vi "BotSpeak.BaseCom.vi"(3 "Termination":string="\r\n", 5 "command":string="PING", 6 "Bot Settings in":T1) -> (0 "response":string="169.254.32.85", 2 "Bot Settings out":T1)   [LabVIEW 2014]
doc: "Protocol:\nLCD \"text to write\" 0,0 // start row, start col (0,0 default)\nBTN // replies with a 5 bit number bot PB1-PB5\nLED 64 // each bit corresponds to an LED\nAI 0 // replies with the value of A/D 0\nAO 2.5,1.34 // sets DAC 0 to 2.5 v and DAC 1 to 1.34 v\nDIO 3,1 // sets DIO 3 to HIGH\nDIO 3 // reads DIO 3 and returns state\nIP // returns IP Address\nTEMP // returns Temperature reading"
uses:
  <userlib>/botspeakLib/VIs/Direct/BotSpeak_Control.ctl
  <userlib>/botspeakLib/VIs/SubVIs/BotSpeak_Globals.vi
panel:
  # "GET DIO[DIO[1]}"
  # "to do:\n\n\nAbort does not work."
  # "use Address \"close\" to close the \nlast connection"
  # "blank means no reply"
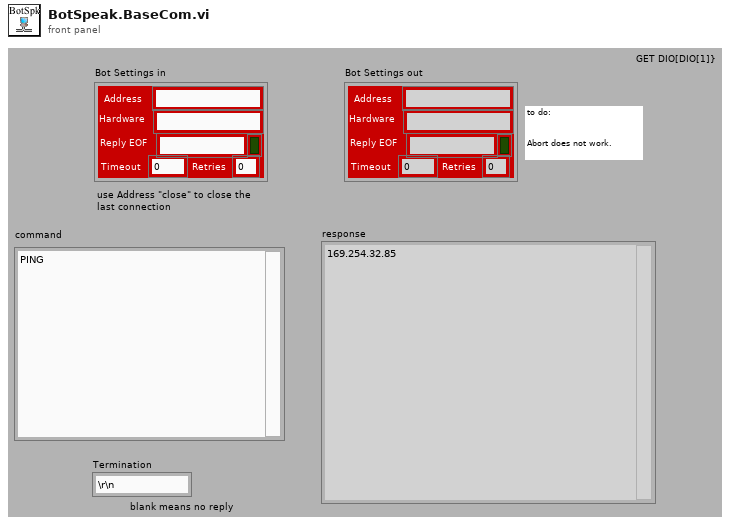
[diagram p1: front panel]
types:
  T1 = typedef "BotSpeak_Control.ctl" = cluster{"Address":string, "Reply EOF":string, "Hardware":string, "Retries":i8, "Timeout":i32, "Open?":bool}
  T2 = typedef "CommState.ctl" = cluster{"Bot Settings":T1, "Initialized":bool, "Talking":bool}
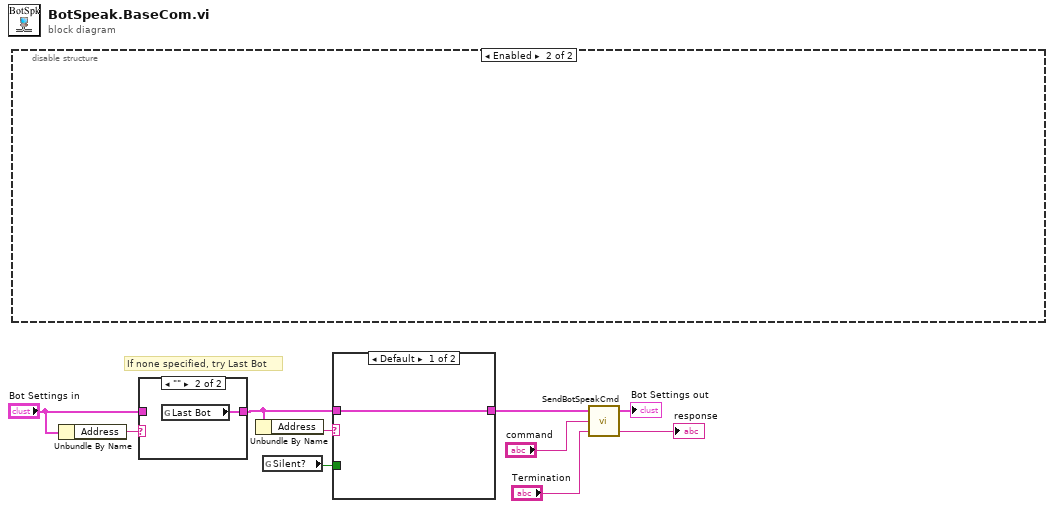
[diagram p0: block diagram]
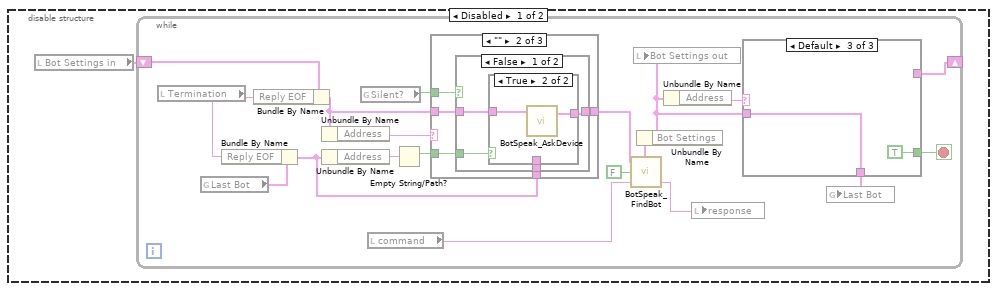
[diagram p2: hidden frame]
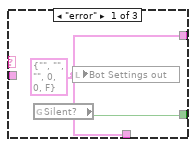
[diagram p3: hidden frame]
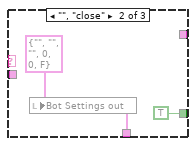
[diagram p4: hidden frame]
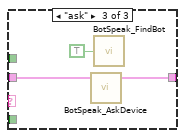
[diagram p8: hidden frame]
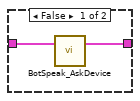
[diagram p10: hidden frame]
diagram:
  # "If none specified, try Last Bot"
  n1 = disable-structure shown="Enabled" {
    frame Disabled {
      n2 = local read "Bot Settings in"() -> (w11:T1)
      n3 = while {
        shift-right: [w17] -> _
        shift-left: w11 -> [w18]
        stop <- w19 stop-if-true
        n4 = local read "Termination"() -> (w15:string)
        n5 = global read "BotSpeak_Globals.vi" "Last Bot"() -> (w24:T1)
        n6 = Bundle By Name(cluster=w24, "Reply EOF"=w15) -> (w23:T1)
        n7 = Bundle By Name(cluster=w18, "Reply EOF"=w15) -> (w27:T1)
        n8 = Unbundle By Name(w27) -> ("Address"=w28:string)
        n9 = Unbundle By Name(w23) -> ("Address"=w30:string)
        n10 = global read "BotSpeak_Globals.vi" "Silent?"() -> (w16:bool)
        n11 = local read "command"() -> (w14:string)
        n12 = Empty String/Path?(string/path=w30) -> (empty?=w29:bool)
        n13 = case shown="\"\"" w28 {
          tunnel: [w37 w41 w52] -> w21
          tunnel: w27 -> [w37 w42 w53]
          tunnel: w29 -> [_ w40 _]
          tunnel: w23 -> [_ w39 _]
          tunnel: w16 -> [_ w38 _]
          frame Default {
          }
          frame "" {
            n14 = case shown="False" w38 {
              tunnel: w42 -> [w46 w50]
              tunnel: [w45 w50] -> w41
              tunnel: w40 -> [w44 _]
              tunnel: w39 -> [w43 _]
              frame False {
                n15 = case shown="True" w44 {
                  tunnel: w46 -> [_ w49]
                  tunnel: [w47 w48] -> w45
                  tunnel: w43 -> [w47 _]
                  frame False {
                  }
                  frame True {
                    n16 = call <userlib>:"BotSpeak_AskDevice.vi"("Bot Settings"=w49) -> ("Bot Settings out"=w48:T1)  [unwired: 2 in]
                  }
                }
              }
              frame True {
              }
            }
          }
          frame "ask" {
            n17 = call <userlib>:"BotSpeak_AskDevice.vi"("Bot Settings"=w53) -> ("Bot Settings out"=w52:T1)  [unwired: 2 in]
            n18 = call <userlib>:"BotSpeak_FindBot.vi"("Reset?"=TRUE) -> ()  [unwired: 2 in, 3 out]
          }
        }
        n19 = call <userlib>:"BotSpeak_FindBot.vi"("String To Send"=w14, "Reset?"=FALSE, "Bot Settings"=w21) -> ("Reply"=w13:string, "Connection"=w20:T2)  [unwired: 1 out]
        n20 = Unbundle By Name(w20) -> ("Bot Settings"=w12:T1)
        n21 = local write "Bot Settings out"(w12) -> ()
        n22 = Unbundle By Name(w12) -> ("Address"=w25:string)
        n23 = local write "response"(w13) -> ()
        n24 = case shown="Default" w25 {
          tunnel: w12 -> [_ _ w36]
          tunnel: [w32 w33 w36] -> w26
          tunnel: [w31 TRUE TRUE] -> w19
          tunnel: [w32 _ _] -> w17
          frame "error" {
            w32 = T1 {"Address"="", "Reply EOF"="", "Hardware"="", "Retries"=0, "Timeout"=0, "Open?"=FALSE} ("Bot Settings Out")
            n25 = global read "BotSpeak_Globals.vi" "Silent?"() -> (w31:bool)
            n26 = local write "Bot Settings out"(w32) -> ()
          }
          frame "", "close" {
            w33 = T1 {"Address"="", "Reply EOF"="", "Hardware"="", "Retries"=0, "Timeout"=0, "Open?"=FALSE} ("Bot Settings Out")
            n27 = local write "Bot Settings out"(w33) -> ()
          }
          frame Default {
          }
        }
        n28 = global write "BotSpeak_Globals.vi" "Last Bot"(w26) -> ()
      }
    }
    frame Enabled {
    }
  }
  n29 = Unbundle By Name("Bot Settings in") -> ("Address"=w10:string)
  n30 = case shown="\"\"" w10 {
    tunnel: [w54 w55] -> w4
    tunnel: "Bot Settings in" -> [w54 _]
    frame Default {
    }
    frame "" {
      n31 = global read "BotSpeak_Globals.vi" "Last Bot"() -> (w55:T1)
    }
  }
  n32 = Unbundle By Name(w4) -> ("Address"=w8:string)
  n33 = global read "BotSpeak_Globals.vi" "Silent?"() -> (w7:bool)
  n34 = case shown="Default" w8 {
    tunnel: w4 -> [w56 w59]
    tunnel: w7 -> [_ w58]
    tunnel: [w56 w57] -> w3
    frame Default {
    }
    frame "", "ask" {
      n35 = case shown="True" w58 {
        tunnel: w59 -> [w61 w62]
        tunnel: [w60 w62] -> w57
        frame False {
          n36 = call <userlib>:"BotSpeak_AskDevice.vi"("Bot Settings"=w61) -> ("Bot Settings out"=w60:T1)  [unwired: 2 in]
        }
        frame True {
        }
      }
    }
  }
  n37 = call <userlib>:"SendBotSpeakCmd.vi"("Termination"="Termination", "command"="command", "Last Bot"=w3) -> ("response"=→"response":string, "Bot Settings out"=→"Bot Settings out":T1)  [unwired: 1 in]
